vi "is valid get request.vi"(11 "first line":string) -> (2 "request URI":string, 3 "valid GET?":bool)   [LabVIEW 2016, in "websocket standalone server.lvclass"]
uses:
  websocket standalone server.lvclass
  <vilib>/Utility/error.llb/whitespace.ctl
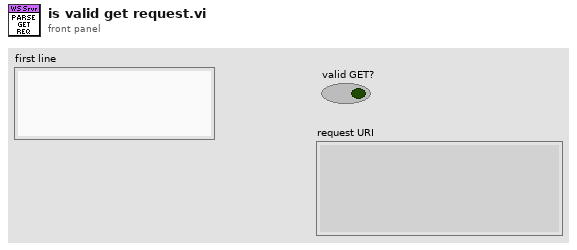
[diagram p1: front panel]
types:
  T1 = typedef "whitespace.ctl" = u16
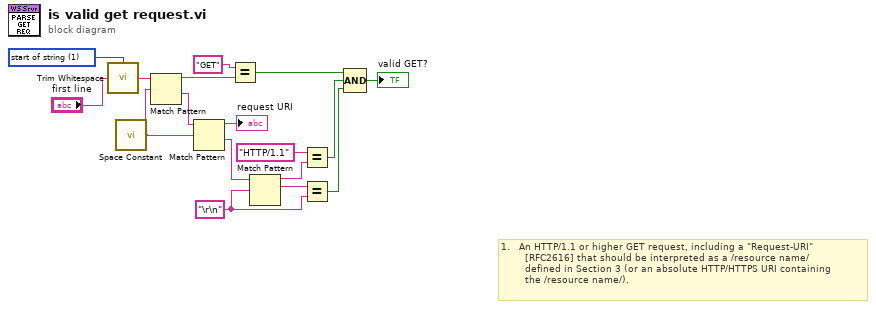
[diagram p0: block diagram]
diagram:
  w11 = T1 1 items=["both", "start of string", "end of string"] ("location (both)")
  w6 = "\r\n"
  # "1.   An HTTP/1.1 or higher GET request, including a \"Request-URI\"\n        [RFC2616] that should be interpreted as a /resource name/\n        defined in Section 3 (or an absolute HTTP/HTTPS URI containing\n        the /resource name/)."
  n1 = call <vilib>:"Trim Whitespace.vi"("string"="first line", "location (both)"=w11) -> ("trimmed string"=w10:string)
  n2 = call <vilib>:"Space Constant.vi"() -> ("String"=w9:string)
  n3 = Match Pattern(string=w10, regular expression=w9) -> (before substring=w15:string, after substring=w7:string)  [unwired: 1 in, 2 out]
  n4 = Match Pattern(string=w7, regular expression=w9) -> (before substring=→"request URI":string, after substring=w8:string)  [unwired: 1 in, 2 out]
  n5 = Equal?(x="GET", y=w15) -> (x = y?=w16:bool)
  n6 = Match Pattern(string=w8, regular expression=w6) -> (before substring=w13:string, match substring=w5:string)  [unwired: 1 in, 2 out]
  n7 = Equal?(x="HTTP/1.1", y=w13) -> (x = y?=w3:bool)
  n8 = Equal?(x=w5, y=w6) -> (x = y?=w2:bool)
  n9 = Compound Arithmetic op=AND(w16, w3, w2) -> (→"valid GET?":bool)
